vi "TestOddEven.vi"(2 "error in (no error)":errorcluster, 3 "Numeric":dbl) -> (0 "error out":errorcluster, 1 "Boolean":bool)   [LabVIEW 2010]
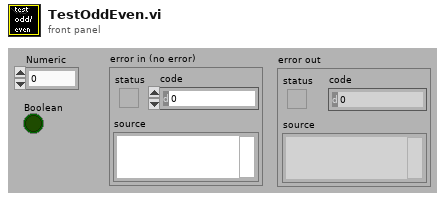
[diagram p1: front panel]
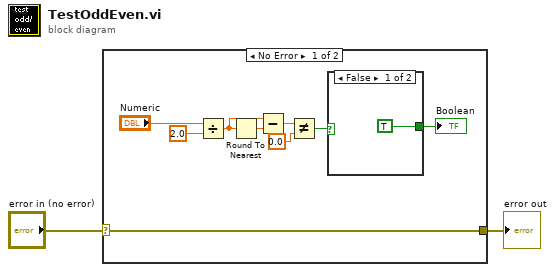
[diagram p0: block diagram]
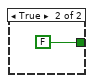
[diagram p2: hidden frame]
diagram:
  n1 = case shown="No Error" "error in (no error)" {
    selector: "error in (no error)" -> [w3 w14]
    tunnel: [w3 w14] -> w1
    frame No Error {
      n2 = Divide(x="Numeric", y=2.0) -> (x/y=w4:dbl)
      n3 = Round To Nearest(number=w4) -> (nearest integer value=w10:dbl)
      n4 = Subtract(x=w4, y=w10) -> (x-y=w8:dbl)
      n5 = Not Equal?(x=w8, y=0.0) -> (x != y?=w6:bool)
      n6 = case shown="False" w6 {
        tunnel: [TRUE FALSE] -> w5
        frame False {
        }
        frame True {
        }
      }
      "Boolean" <- w5
    }
    frame Error {
    }
  }
  "error out" <- w1
